vi "Execution Unit.Async.vi"(10 "Parameters":variant, 11 "Process":refnum<class "Process.lvclass">) -> ()   [LabVIEW 2020, in "Communication Bus Template Engine.lvlib" / "Custom Device.lvlib"]
uses:
  Custom Device.lvlib
  <vilib>/NI/NIVS Inline Async API/_VS Inline Async API/Process/Process.lvclass
  Asynchronous Process Parameters.ctl
  Asynchronous Execution Unit Runtime Information.ctl
  Interfaces/Execution Unit/Execution Unit.lvclass
  Interfaces/Shared Resources/Shared Resources.lvclass
  <vilib>/NI/NIVS Inline Async API/_VS Inline Async API/Process/Process.lvclass/Process.ctl
  <vilib>/NI/NIVS Inline Async API/_Data Access Engine/Access Type Classes/ReadWrite/ReadWrite.lvclass/ReadWrite.ctl
  <vilib>/NI/NIVS Inline Async API/_Data Access Engine/Access Type Classes/Read/Read.lvclass/Read.ctl
  <vilib>/NI/NIVS Inline Async API/_Data Access Engine/Access Type Classes/Write/Write.lvclass/Write.ctl
  <vilib>/NI/NIVS Inline Async API/_Data Access Engine/Data Access Engine/Methods/Read.Data.vi
  <vilib>/NI/NIVS Inline Async API/_Data Access Engine/Data Access Engine/Methods/Write.Data.vi
  <vilib>/NI/NIVS Inline Async API/_Data Access Engine/Data Access Engine/Methods/ReadWrite.Data.vi
  <vilib>/NI/NIVS Inline Async API/_Data Access Engine/Data Access Engine/Methods/ReadWrite.Data.Reset.vi
  <vilib>/NI/NIVS Inline Async API/_VS Inline Async API/Process/Data Member Access/Read Data Access.vi
  <vilib>/NI/NIVS Inline Async API/_VS Inline Async API/Error Handling Process/SubVIs/Error.ConvertArray.vi
  <vilib>/NI/NIVS Inline Async API/_Data Access Engine/Access Type Classes/Read/Read.ProcessData.vi
  <vilib>/NI/NIVS Inline Async API/_Data Access Engine/Access Type Classes/Write/Write.ProcessData.vi
  <vilib>/NI/NIVS Inline Async API/_Data Access Engine/Access Type Classes/ReadWrite/ReadWrite.ProcessData.vi
  <vilib>/NI/NIVS Inline Async API/_Data Access Engine/Access Type Classes/ReadWrite/ReadWrite.ProcessData.Reset.vi
  <vilib>/NI/NIVS Inline Async API/_Data Access Engine/Access Type Classes/Write/Write.Buffer.vi
  <vilib>/NI/NIVS Inline Async API/_Data Access Engine/Access Type Classes/Write/Write.Commit.vi
  <vilib>/NI/NIVS Inline Async API/_Data Access Engine/Data Access Engine/Methods/Write.Lookup.vi
  <vilib>/NI/NIVS Inline Async API/_Data Access Engine/Data Access Engine/Methods/ReadWrite.Lookup.vi
  <vilib>/NI/NIVS Inline Async API/_Data Access Engine/Data Access Engine/Methods/Read.Lookup.vi
  <vilib>/NI/NIVS Inline Async API/_Data Access Engine/Data Access Engine/Data Access Engine.lvclass
  <vilib>/NI/NIVS Inline Async API/_Data Access Engine/Access Type Classes/ReadWrite/ReadWrite.lvclass
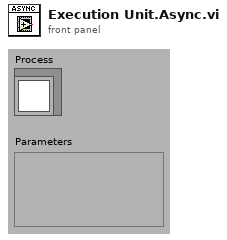
[diagram p1: front panel]
types:
  T1 = typedef "Communication Bus Template Engine.lvlib/Custom Device.lvlib/Asynchronous Process Parameters.ctl" = cluster{"Asynchronous Execution Unit Runtime Information":T2, "shared resources":refnum<class "Shared Resources.lvclass">}
  T2 = typedef "Communication Bus Template Engine.lvlib/Custom Device.lvlib/Asynchronous Execution Unit Runtime Information.ctl" = cluster{"Execution Unit":refnum<class "Execution Unit.lvclass">, "Incoming Channel Group Name":string, "Outgoing Channel Group Name":string, "ReadWrite Channel Group Name":string}
  T3 = typedef "Data Access Engine.lvlib/Data Access Engine.lvclass/Write.DVR.ctl" = refnum<data-value>
  T4 = typedef "Data Access Engine.lvlib/Data Access Engine.lvclass/ReadWrite.DVR.ctl" = refnum<data-value>
  T5 = typedef "Data Access Engine.lvlib/Data Access Engine.lvclass/Read.DVR.ctl" = refnum<data-value>
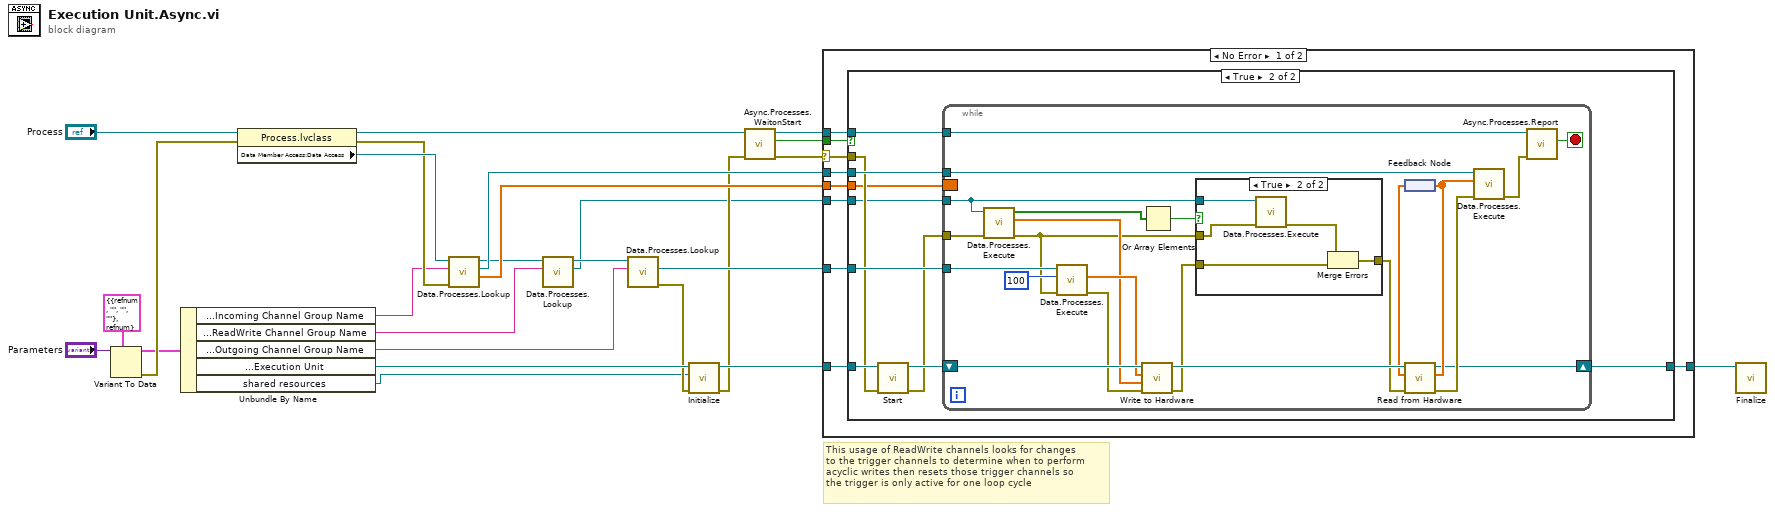
[diagram p0: block diagram]
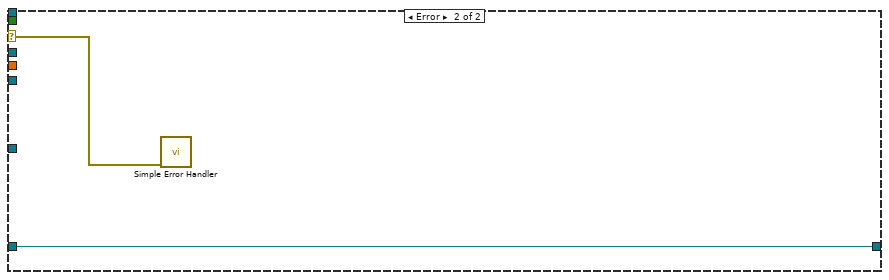
[diagram p4: hidden frame]
diagram:
  # "This usage of ReadWrite channels looks for changes\nto the trigger channels to determine when to perform\nacyclic writes then resets those trigger channels so\nthe trigger is only active for one loop cycle"
  n1 = Variant To Data(type=T1 {"Asynchronous Execution Unit Runtime Information"={"Execution Unit"=refnum, "Incoming Channel Group Name"="", "Outgoing Channel Group Name"="", "ReadWrite Channel Group Name"=""}, "shared resources"=refnum} ("Asynchronous Process Parameters"), Variant="Parameters") -> (data=w14:T1, error out=w15:errorcluster)  [unwired: 1 in]
  n2 = Unbundle By Name(w14) -> ("Asynchronous Execution Unit Runtime Information.Incoming Channel Group Name"=w5:string, "Asynchronous Execution Unit Runtime Information.ReadWrite Channel Group Name"=w4:string, "Asynchronous Execution Unit Runtime Information.Outgoing Channel Group Name"=w13:string, "Asynchronous Execution Unit Runtime Information.Execution Unit"=w11:refnum<class "Execution Unit.lvclass">, "shared resources"=w6:refnum<class "Shared Resources.lvclass">)
  n3 = property class="Process.lvclass"(reference="Process", error in=w15) -> (reference out=w20:refnum<class "Process.lvclass">, error out=w18:errorcluster, "Data Member Access:Data Access"=w19:refnum<class "Data Access Engine.lvclass">)
  n4 = call-poly <vilib>:"Data.Processes.Lookup.vi"("error in (no error)"=w18, "Name"=w5, "Data Access API in"=w19) -> ("Initial Values"=w12:dbl[], "Ref"=w22:T3, "Data Access API out"=w3:refnum<class "Data Access Engine.lvclass">)  [unwired: 5 in, 1 out]
  n5 = call-poly <vilib>:"Data.Processes.Lookup.vi"("Name"=w4, "Data Access API in"=w3) -> ("Ref"=w1:T4, "Data Access API out"=w2:refnum<class "Data Access Engine.lvclass">)  [unwired: 6 in, 2 out]
  n6 = call-poly <vilib>:"Data.Processes.Lookup.vi"("Name"=w13, "Data Access API in"=w2) -> ("error out"=w9:errorcluster, "Ref"=w23:T5)  [unwired: 6 in, 2 out]
  n7 = call-dynamic "Initialize.vi"("error in (no error)"=w9, "shared resources"=w6, "Execution Unit in"=w11) -> ("error out"=w8:errorcluster, "Execution Unit out"=w10:refnum<class "Execution Unit.lvclass">)  [unwired: 7 in]
  n8 = call <vilib>:"Async.Processes.WaitonStart.vi"("error in (no error)"=w8, "Process"=w20) -> ("error out"=w24:errorcluster, "Execute"=w26:bool, "Process out"=w25:refnum<class "Process.lvclass">)  [unwired: 7 in]
  n9 = case shown="No Error" w24 {
    selector: w24 -> [w31 w76]
    tunnel: w26 -> [w35 _]
    tunnel: w25 -> [w34 _]
    tunnel: w22 -> [w33 _]
    tunnel: w23 -> [w32 _]
    tunnel: w12 -> [w30 _]
    tunnel: w10 -> [w29 w75]
    tunnel: [w28 w75] -> w7
    tunnel: w1 -> [w27 _]
    frame No Error {
      n10 = case shown="True" w35 {
        tunnel: w31 -> [_ w42]
        tunnel: w34 -> [_ w44]
        tunnel: w32 -> [_ w46]
        tunnel: w33 -> [_ w45]
        tunnel: w30 -> [_ w40]
        tunnel: w29 -> [w36 w43]
        tunnel: [w36 w39] -> w28
        tunnel: w27 -> [_ w38]
        frame False {
        }
        frame True {
          n11 = call-dynamic "Start.vi"("error in (no error)"=w42, "Execution Unit in"=w43) -> ("error out"=w37:errorcluster, "Execution Unit out"=w41:refnum<class "Execution Unit.lvclass">)  [unwired: 8 in]
          n12 = while {
            tunnel: w44 -> [w68]
            tunnel: w46 -> [w66]
            tunnel: w45 -> [w65]
            border: w40 -> [_]
            shift-right: [w55] -> w39
            shift-left: w41 -> [w63]
            tunnel: w38 -> [w54]
            tunnel: w37 -> [w53]
            stop <- w67 stop-if-true
            n13 = call-poly <vilib>:"Data.Processes.Execute.vi"("error in (no error)"=w53, "Ref"=w54) -> ("error out"=w49:errorcluster, "Data"=w52:dbl[], "Detect?"=w51:bool[])  [unwired: 6 in, 1 out]
            n14 = call-poly <vilib>:"Data.Processes.Execute.vi"("error in (no error)"=w49, "timeout ms"=100, "Ref"=w66) -> ("error out"=w60:errorcluster, "Values"=w61:dbl[])  [unwired: 6 in, 1 out]
            n15 = call-dynamic "Write to Hardware.vi"("error in (no error)"=w60, "Trigger Values"=w52, "Values in"=w61, "Execution Unit in"=w63) -> ("error out"=w48:errorcluster, "Execution Unit out"=w62:refnum<class "Execution Unit.lvclass">)  [unwired: 4 in, 2 out]
            n16 = Or Array Elements(Boolean array=w51) -> (logical OR=w50:bool)
            n17 = case shown="True" w50 {
              tunnel: w54 -> [_ w74]
              tunnel: w49 -> [_ w72]
              tunnel: w48 -> [w69 w73]
              tunnel: [w69 w70] -> w47
              frame False {
              }
              frame True {
                n18 = call-poly <vilib>:"Data.Processes.Execute.vi"("error in (no error)"=w72, "Ref"=w74) -> ("error out"=w71:errorcluster)  [unwired: 8 in, 1 out]
                n19 = Merge Errors(w71, w73) -> (w70:errorcluster)
              }
            }
            n20 = feedback #1() -> (w57:dbl[])
            n21 = call-dynamic "Read from Hardware.vi"("error in (no error)"=w47, "Values in"=w57, "Execution Unit in"=w62) -> ("error out"=w59:errorcluster, "Values out"=w56:dbl[], "Execution Unit out"=w55:refnum<class "Execution Unit.lvclass">)  [unwired: 6 in]
            n22 = feedback-in #1(w56) -> ()
            n23 = call-poly <vilib>:"Data.Processes.Execute.vi"("error in (no error)"=w59, "Values"=w56, "Ref"=w65) -> ("error out"=w58:errorcluster)  [unwired: 8 in]
            n24 = call <vilib>:"Async.Processes.Report.vi"("Error"=w58, "Process in"=w68) -> ("Stop"=w67:bool)  [unwired: 8 in, 1 out]
          }
        }
      }
    }
    frame Error {
      n25 = call <vilib>:"Simple Error Handler.vi"("error in (no error)"=w76) -> ()  [unwired: 4 in, 5 out]
    }
  }
  n26 = call-dynamic "Finalize.vi"("Execution Unit in"=w7) -> ()  [unwired: 9 in, 2 out]
